vi "Get PDO Communication Parmameter.vi"(8 "error in (no error)":errorcluster, 11 "PDO Slot in":refnum<class "PDO Slot.lvclass">) -> (0 "error out":errorcluster, 2 "PDO Grid.lvlib:PDO Communication Parameter":refnum<class "PDO Communication Parameter.lvclass">, 3 "PDO Slot out":refnum<class "PDO Slot.lvclass">)   [LabVIEW 2019, in "PDO Grid.lvlib" / "PDO Slot.lvclass"]
uses:
  PDO Slot.lvclass
  PDO Slot.lvclass/PDO Slot.ctl
  Core/PDO Communication Parameter/PDO Communication Parameter.lvclass
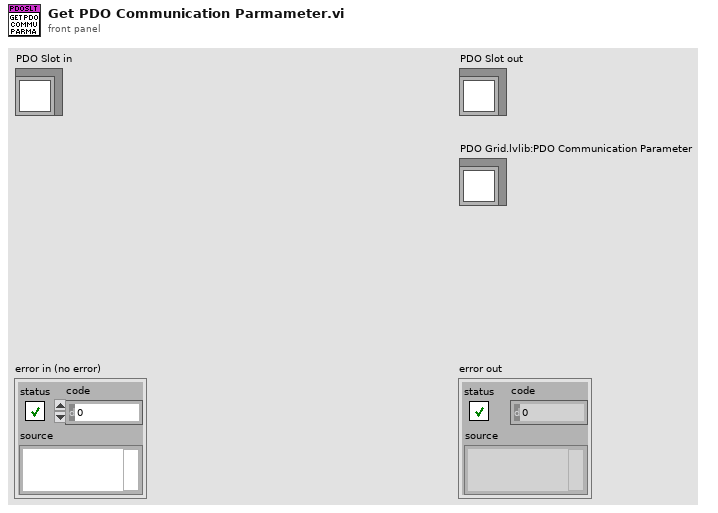
[diagram p1: front panel]
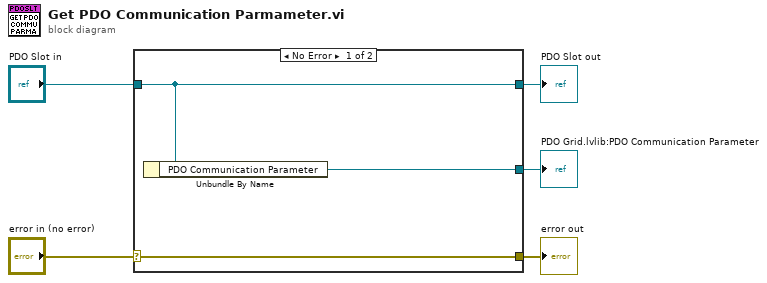
[diagram p0: block diagram]
diagram:
  n1 = case shown="No Error" "error in (no error)" {
    selector: "error in (no error)" -> [w8 w9]
    tunnel: [w8 w9] -> w4
    tunnel: [w7 w10] -> w2
    tunnel: "PDO Slot in" -> [w7 w10]
    tunnel: [w6 _] -> w1
    frame No Error {
      n2 = Unbundle By Name(w7) -> ("PDO Communication Parameter"=w6:refnum<class "PDO Communication Parameter.lvclass">)
    }
    frame Error {
    }
  }
  "error out" <- w4
  "PDO Slot out" <- w2
  "PDO Grid.lvlib:PDO Communication Parameter" <- w1
